vi "HighpassFilter.vi"(8 "error in (no error)":errorcluster, 10 "Integration Properties in":T1={"Conversion Op"=enum."singleInt", "Unit"="", "Parent Unit"="", "Single Integration Cutoff"=0.0, "Double Integration Cutoff"=0.0, "Lowpass Filter State"={"designed"=FALSE, "integration filter coefficients"={"beta"=0.0, "gamma"=0.0, "alpha"=0.0}, "state"={"x(n-1) state"=0.0, "y(n-1) state"=0.0, "x(n-2) state"=0.0, "y(n-2) state"=0.0}}, "Highpass Filter State"={"designed"=FALSE, "IIR Filter Cluster"={"filter structure"=enum."IIR 2nd Order", "Reverse Coefficients"=[], "Forward Coefficients"=[]}, "Filter State"=[]}, "Wfm Scale"=0.0} {"Highpass Filter State"."Filter State" format="%.2f"; "Highpass Filter State"."IIR Filter Cluster"."Forward Coefficients" format="%.2f"; "Highpass Filter State"."IIR Filter Cluster"."Reverse Coefficients" format="%.2f"; "Lowpass Filter State"."state"."y(n-2) state" format="%.2f"; "Lowpass Filter State"."state"."x(n-2) state" format="%.2f"; "Lowpass Filter State"."state"."y(n-1) state" format="%.2f"; "Lowpass Filter State"."state"."x(n-1) state" format="%.2f"}, 11 "Waveform":waveform(sgl)) -> (0 "error out":errorcluster, 2 "Integration Properties out":T1={"Conversion Op"=enum."singleInt", "Unit"="", "Parent Unit"="", "Single Integration Cutoff"=0.0, "Double Integration Cutoff"=0.0, "Lowpass Filter State"={"designed"=FALSE, "integration filter coefficients"={"beta"=0.0, "gamma"=0.0, "alpha"=0.0}, "state"={"x(n-1) state"=0.0, "y(n-1) state"=0.0, "x(n-2) state"=0.0, "y(n-2) state"=0.0}}, "Highpass Filter State"={"designed"=FALSE, "IIR Filter Cluster"={"filter structure"=enum."IIR 2nd Order", "Reverse Coefficients"=[], "Forward Coefficients"=[]}, "Filter State"=[]}, "Wfm Scale"=0.0} {"Highpass Filter State"."Filter State" format="%.2f"; "Highpass Filter State"."IIR Filter Cluster"."Forward Coefficients" format="%.2f"; "Highpass Filter State"."IIR Filter Cluster"."Reverse Coefficients" format="%.2f"; "Lowpass Filter State"."state"."y(n-2) state" format="%.2f"; "Lowpass Filter State"."state"."x(n-2) state" format="%.2f"; "Lowpass Filter State"."state"."y(n-1) state" format="%.2f"; "Lowpass Filter State"."state"."x(n-1) state" format="%.2f"}, 3 "Highpass Filtered Waveform":waveform(sgl))   [LabVIEW 2017, in "CmsVirtualChannel.lvlib"]
uses:
  <vilib>/addons/InsightCM/Devices/Shared/Cms/CmsVirtualChannel/CmsVirtualChannel.lvlib
  <vilib>/addons/InsightCM/Devices/Shared/Cms/CmsVirtualChannel/controls/Integration.ctl
  <vilib>/addons/InsightCM/Utilities/Analysis/Shared/controls/ConversionOp.ctl
  <vilib>/addons/InsightCM/Utilities/Analysis/Vibration/controls/LowPassFilterState.ctl
  <vilib>/addons/InsightCM/Utilities/Analysis/Vibration/controls/HighPassFilterState.ctl
  <vilib>/addons/InsightCM/Utilities/Analysis/Vibration/VibrationAnalysisFunctions.lvlib
  <vilib>/addons/InsightCM/Utilities/Analysis/Shared/AnalysisHelper.lvlib
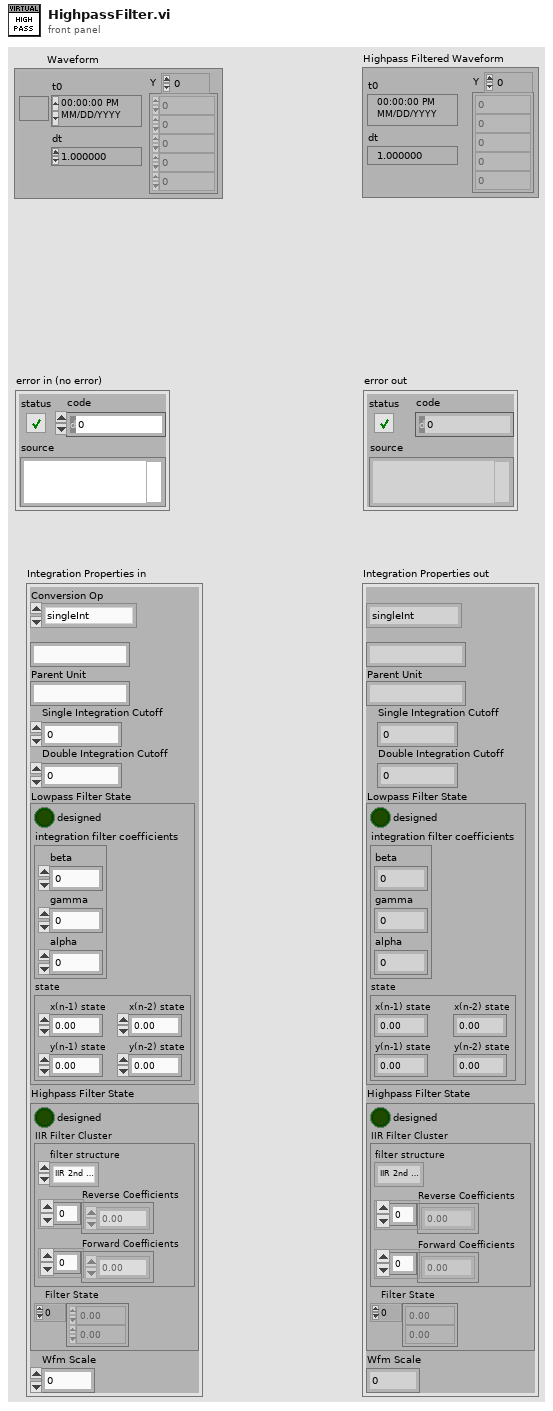
[diagram p1: front panel]
types:
  T1 = typedef "CmsVirtualChannel.lvlib/Integration.ctl" = cluster{"Conversion Op":T2, "Unit":string, "Parent Unit":string, "Single Integration Cutoff":dbl, "Double Integration Cutoff":dbl, "Lowpass Filter State":T3, "Highpass Filter State":T4, "Wfm Scale":sgl}
  T2 = typedef "AnalysisHelper.lvlib/ConversionOp.ctl" = enum16{"none", "singleInt", "doubleInt", "singleDiff", "doubleDiff"}
  T3 = typedef "VibrationAnalysisFunctions.lvlib/LowPassFilterState.ctl" = cluster{"designed":bool, "integration filter coefficients":cluster{"beta":dbl, "gamma":dbl, "alpha":dbl}, "state":cluster{"x(n-1) state":dbl, "y(n-1) state":dbl, "x(n-2) state":dbl, "y(n-2) state":dbl}}
  T4 = typedef "VibrationAnalysisFunctions.lvlib/HighPassFilterState.ctl" = cluster{"designed":bool, "IIR Filter Cluster":cluster{"filter structure":enum32{"IIR 2nd Order", "IIR 4th Order"}, "Reverse Coefficients":dbl[], "Forward Coefficients":dbl[]}, "Filter State":dbl[]}
  T5 = cluster{"filter structure":enum32{"IIR 2nd Order", "IIR 4th Order"}, "Reverse Coefficients":dbl[], "Forward Coefficients":dbl[]}
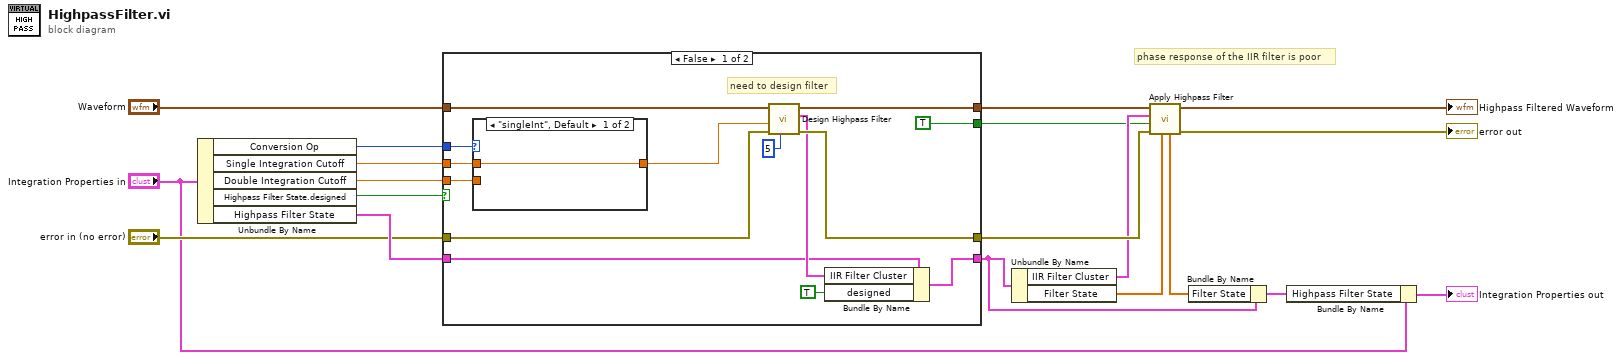
[diagram p0: block diagram]
diagram:
  # "phase response of the IIR filter is poor"
  n1 = Unbundle By Name("Integration Properties in") -> ("Conversion Op"=w1:T2, "Single Integration Cutoff"=w6:dbl, "Double Integration Cutoff"=w5:dbl, "Highpass Filter State.designed"=w12:bool, "Highpass Filter State"=w11:T4)
  n2 = case shown="False" w12 {
    tunnel: "error in (no error)" -> [w20 w37]
    tunnel: "Waveform" -> [w33 w38]
    tunnel: [w31 w38] -> w16
    tunnel: [w30 w37] -> w17
    tunnel: w11 -> [w27 w36]
    tunnel: [w28 w36] -> w8
    tunnel: [TRUE ("reset") _] -> w13
    tunnel: w1 -> [w24 _]
    tunnel: w6 -> [w22 _]
    tunnel: w5 -> [w21 _]
    frame False {
      # "need to design filter"
      n3 = case shown="\"singleInt\", Default" w24 {
        tunnel: [w34 w35] -> w23
        tunnel: w22 -> [w34 _]
        tunnel: w21 -> [_ w35]
        frame "singleInt", Default {
        }
        frame "doubleInt" {
        }
      }
      n4 = call <vilib>:"Design Highpass Filter.vi"("highpass filter order"=5, "error in (no error)"=w20, "highpass cutoff frequency"=w23, "input signal"=w33) -> ("error out"=w30:errorcluster, "IIR Filter Cluster"=w29:T5, "dup signal"=w31:waveform(sgl))  [unwired: 5 in]
      n5 = Bundle By Name(cluster=w27, "IIR Filter Cluster"=w29, "designed"=TRUE) -> (w28:T4)
    }
    frame True {
      # "filter already designed"
    }
  }
  n6 = Unbundle By Name(w8) -> ("IIR Filter Cluster"=w15:T5, "Filter State"=w14:dbl[])
  n7 = call <vilib>:"Apply Highpass Filter.vi"("Initial Filter State"=w14, "error in (no error)"=w17, "init/cont (init:F)"=w13, "filter coefficients"=w15, "signal [V]"=w16) -> ("error out"=→"error out":errorcluster, "filtered signal [EU]"=→"Highpass Filtered Waveform":waveform(sgl), "Final Filter State"=w9:dbl[])  [unwired: 4 in]
  n8 = Bundle By Name(cluster=w8, "Filter State"=w9) -> (w4:T4)
  n9 = Bundle By Name(cluster="Integration Properties in", "Highpass Filter State"=w4) -> (→"Integration Properties out":T1)
